vi "Get Name.vi"(8 "error in (no error)":errorcluster, 11 "MemberInfo in":refnum<class "Information.lvclass">) -> (0 "error out":errorcluster, 2 "学号(\"\")":string, 3 "MemberInfo out":refnum<class "Information.lvclass">)   [LabVIEW 2015, in "Information.lvclass"]
uses:
  Information.lvclass
  Information.lvclass/Information.ctl
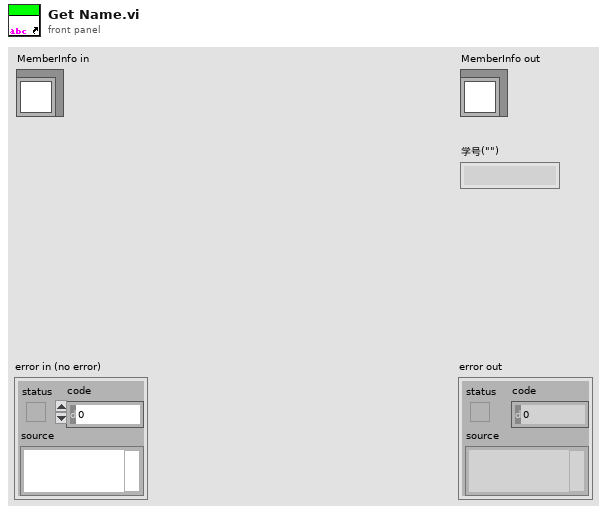
[diagram p1: front panel]
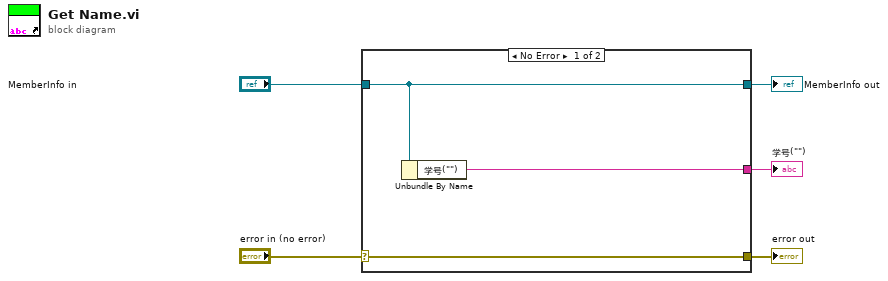
[diagram p0: block diagram]
diagram:
  n1 = case shown="No Error" "error in (no error)" {
    selector: "error in (no error)" -> [w8 w9]
    tunnel: [w8 w9] -> w4
    tunnel: [w7 w10] -> w2
    tunnel: "MemberInfo in" -> [w7 w10]
    tunnel: [w6 _] -> w1
    frame No Error {
      n2 = Unbundle By Name(w7) -> ("学号(\"\")"=w6:string)
    }
    frame Error {
    }
  }
  "error out" <- w4
  "MemberInfo out" <- w2
  "学号(\"\")" <- w1
